vi "Data_Generation.vi"() -> ()   [LabVIEW 2020]
uses:
  <vilib>/Utility/NIReport.llb/Report Type.ctl
  <vilib>/addons/_office/excel.llb/Excel Easy Table (num).vi
  <vilib>/Utility/NIReport.llb/NI_report.lvclass
  <vilib>/addons/_office/NI_ReportGenerationToolkit.lvlib
  <vilib>/Utility/NIReport.llb/NI_ReportGenerationCore.lvlib
  <vilib>/Utility/NIReport.llb/Excel/NI_Excel.lvclass
panel:
  out "error out":errorcluster
  in  "OK Button":bool
  in  "Voltages Header Array":dbl[](array[numeric])
  in  "VISA resource name":refnum<visa-resource-name>
  in  "error in (no error)":errorcluster
  # "0, 0.1, 0.2, 0.3, 0.4, 0.5, 0.7, 1, 2, 3, 4, 5, 7, 10"
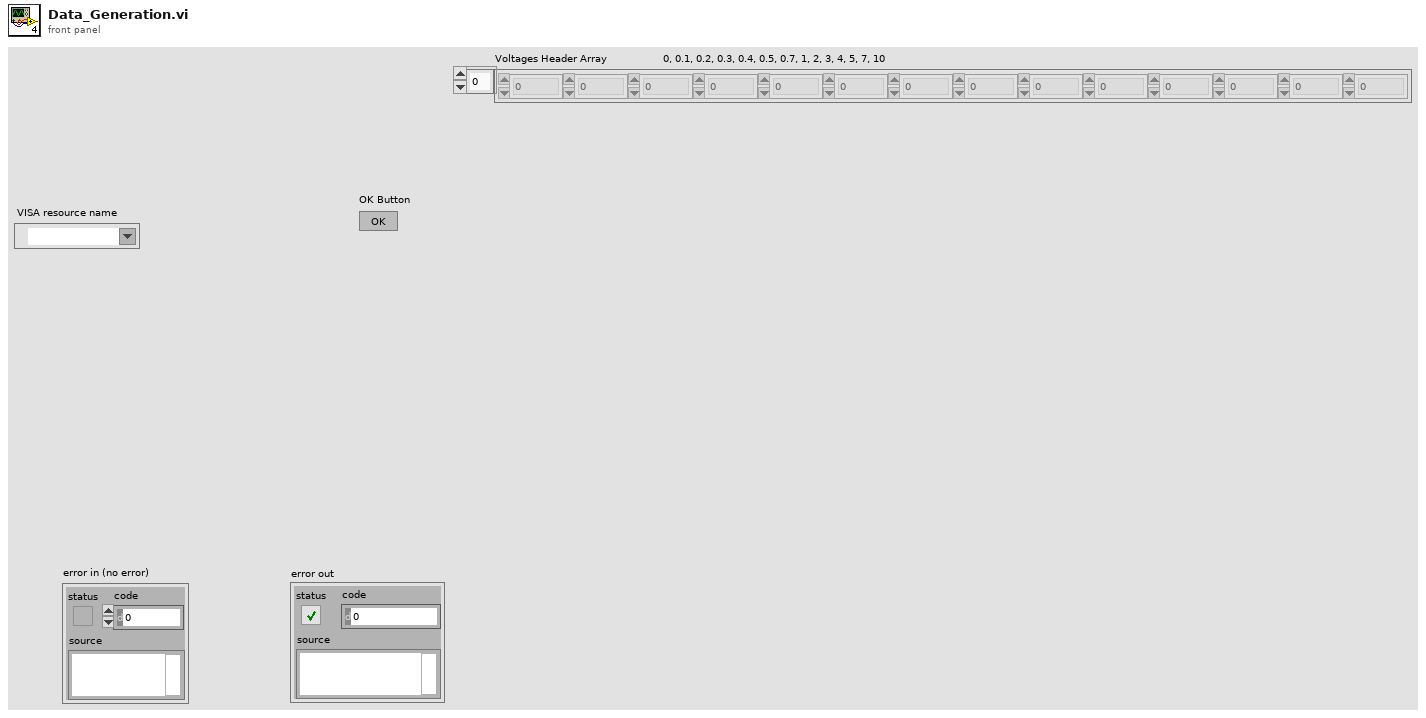
[diagram p1: front panel]
types:
  T1 = typedef "NI_ReportGenerationCore.lvlib/Report Type.ctl" = enum16{"HTML", "Word", "Excel"}
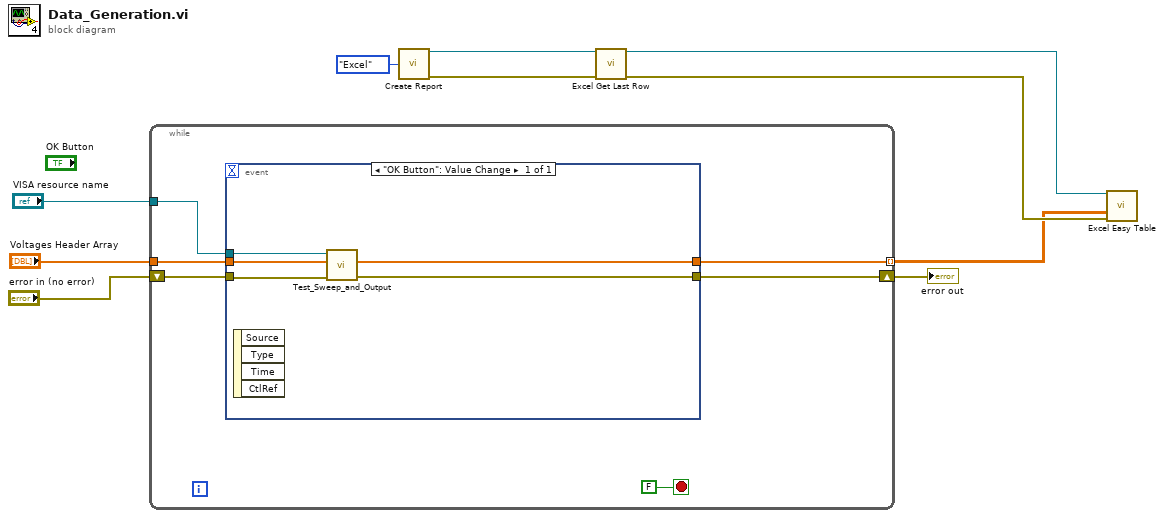
[diagram p0: block diagram]
diagram:
  n1 = while {
    tunnel: "VISA resource name" -> [w12]
    shift-right: [w15] -> w8
    shift-left: "error in (no error)" -> [w16]
    tunnel: "Voltages Header Array" -> [w13]
    tunnel: [w11] -> w1 mode=indexing
    stop <- FALSE stop-if-true
    n2 = event shown="[0] \"OK Button\": Value Change" {
      selector: _ -> [_]
      dyn-events: _ -> [_]
      timeout: _ -> [_]
      tunnel: w16 -> [w21]
      tunnel: [w20] -> w15
      tunnel: w13 -> [w18]
      tunnel: w12 -> [w19]
      tunnel: [w17] -> w11
      event "OK Button": Value Change {
        n3 = event-data() -> ()  [unwired: 1 in, 4 out]
        n4 = call "Test_Sweep_and_Output.vi"("error in (no error)"=w21, "element"=w18, "VISA resource name"=w19) -> ("error out"=w20:errorcluster, "Results_Array"=w17:dbl[])  [unwired: 7 in]
      }
    }
  }
  "error out" <- w8
  n5 = call <vilib>:"Create Report.vi"("report type"=Report_Type."Excel") -> ("report out"=w3:refnum<class "NI_report.lvclass">, "error out"=w2:errorcluster)  [unwired: 13 in]
  n6 = call <vilib>:"Excel Get Last Row.vi"("report in"=w3, "error in (no error)"=w2) -> ("report out"=w5:refnum<class "NI_report.lvclass">, "error out"=w4:errorcluster)  [unwired: 11 in, 1 out]
  n7 = call-poly <vilib>:"Excel Easy Table.vi"("report in"=w5, "text data"=w1, "error in (no error)"=w4) -> ()  [unwired: 8 in, 5 out]
